vi "Example5a.vi"() -> ()   [LabVIEW 2019]
panel:
  out "Triggered":bool
  in  "Threshold":dbl
  in  "Slide":dbl(slide) scale=0.0..10.0
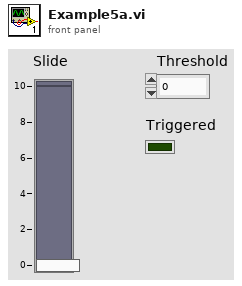
[diagram p1: front panel]
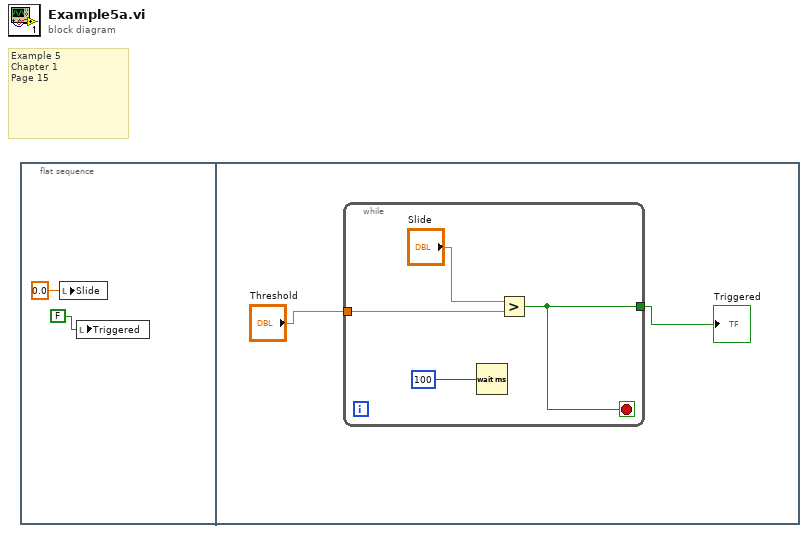
[diagram p0: block diagram]
diagram:
  # "Example 5\nChapter 1\nPage 15"
  n1 = flat-sequence {
    frame #0 {
      n2 = local write "Slide"(0.0 ("Slide")) -> ()
      n3 = local write "Triggered"(FALSE ("Triggered")) -> ()
    }
    frame #1 {
      n4 = while {
        tunnel: [w6] -> w3
        tunnel: "Threshold" -> [w5]
        stop <- w6 stop-if-true
        n5 = Wait (ms)(milliseconds to wait=u32 100) -> ()  [unwired: 1 out]
        n6 = Greater?(x="Slide", y=w5) -> (0:w6:bool)
      }
      "Triggered" <- w3
    }
  }
